vi "Insert_into_Map.vi"(0 "Object_Data_In":T2, 1 "Create_Second_Key (T)":bool=TRUE, 2 "First_Action":T1=enum."Add or Modify Entry", 5 "First_Key":string, 7 "Second_Key":string, 9 "Calculator.lvclass":refnum<class "Calculator.lvclass">, 11 "Error_In":errorcluster, 13 "Second_Action":T1) -> (4 "Object_Data_Out":T2, 6 "Second_Key":string, 15 "error out":errorcluster)   [LabVIEW 2021]
doc: "Used to insert the elements into the map"
uses:
  <vilib>/Utility/miscctls.llb/LVMapReplaceAction.ctl
  Classes/Calculator/Calculator.lvclass
  Controls/Object_Data.ctl
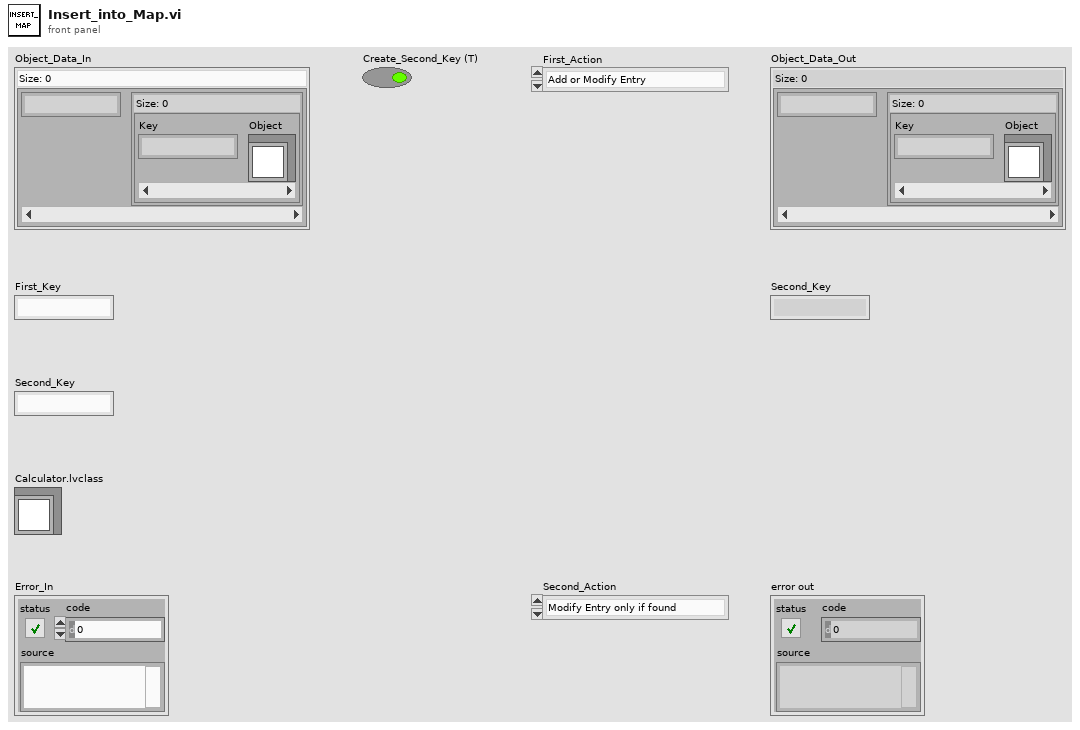
[diagram p1: front panel]
types:
  T1 = typedef "LVMapReplaceAction.ctl" = enum32{"Modify Entry only if found", "Add or Modify Entry", "Delete Entry"}
  T2 = typedef "Object_Data.ctl" = map{string, map{string, refnum<class "Calculator.lvclass">}}
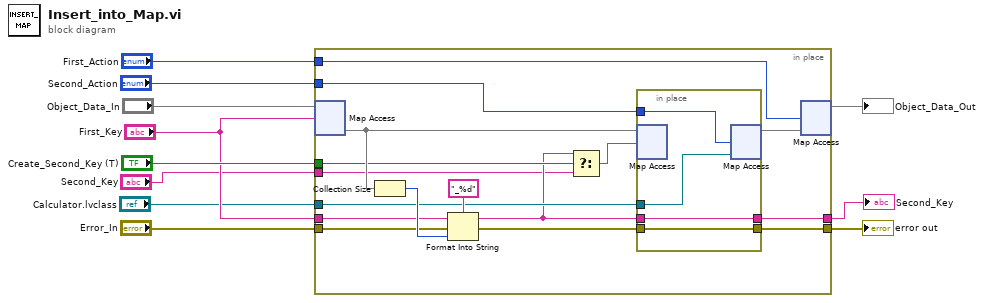
[diagram p0: block diagram]
diagram:
  n1 = in-place {
    in-place-border: "Error_In" -> [w25]
    in-place-border: [w22] -> w11
    in-place-border: "Calculator.lvclass" -> [w20]
    in-place-border: "First_Key" -> [w19]
    in-place-border: [w18] -> w9
    in-place-border: "First_Action" -> [w17]
    in-place-border: "Create_Second_Key (T)" -> [w16]
    in-place-border: "Second_Key" -> [w13]
    in-place-border: "Second_Action" -> [w12]
    n2 = in-place-map #1("Object_Data_In", "First_Key") -> (w23:map{string, refnum<class "Calculator.lvclass">})  [unwired: 1 in, 1 out]
    n3 = Collection Size(1:w23) -> (0:w27:i32)
    n4 = Format Into String(format string="_%d", initial string=w19, error in=w25, w27) -> (resulting string=w14:string, error out=w24:errorcluster)
    n5 = Select(t=w14, s=w16, f=w13) -> (s? t:f=w15:string)
    n6 = in-place {
      in-place-border: w24 -> [w31]
      in-place-border: [w31] -> w22
      in-place-border: w20 -> [w30]
      in-place-border: [w29] -> w18
      in-place-border: w14 -> [w29]
      in-place-border: w12 -> [w28]
      n7 = in-place-map #2(w23, w15) -> ()  [unwired: 1 in, 2 out]
      n8 = in-place-map #2(w30, w28) -> (w21:map{string, refnum<class "Calculator.lvclass">})  [unwired: 2 out]
    }
    n9 = in-place-map #1(w21, w17) -> (→"Object_Data_Out":T2)  [unwired: 2 out]
  }
  "error out" <- w11
  "Second_Key" <- w9
